vi "Supplementary Fig.15.vi"() -> ()   [LabVIEW 2018]
uses:
  <vilib>/Utility/miscctls.llb/LVBoundsTypeDef.ctl
  <vilib>/Analysis/baseanly.llb/Mean (DBL).vi
  <vilib>/Analysis/NI_AALBase.lvlib
panel:
  out "files":string[](array[string])=["3rd-no3_th0_20191112171700-ext.FIRE", "3rd-no3_th0_20191112171706-ext.FIRE", "3rd-no3_th0_20191112171712-ext.FIRE", "3rd-no3_th0_20191112171717-ext.FIRE", "3rd-no3_th0_20191112171723-ext.FIRE", "3rd-no3_th0_20191112171728-ext.FIRE", "3rd-no3_th0_20191112171733-ext.FIRE", "3rd-no3_th0_20191112171739-ext.FIRE", "3rd-no3_th0_20191112171744-ext.FIRE", "3rd-no3_th0_20191112171750-ext.FIRE", "3rd-no3_th0_20191112171756-ext.FIRE", "3rd-no3_th0_20191112171801-ext.FIRE", "3rd-no3_th0_20191112171807-ext.FIRE", "3rd-no3_th0_20191112171813-ext.FIRE", "3rd-no3_th0_20191112171819-ext.FIRE", "3rd-no3_th0_20191112171824-ext.FIRE", "3rd-no3_th0_20191112171829-ext.FIRE", "3rd-no3_th0_20191112171835-ext.FIRE", "3rd-no3_th0_20191112171840-ext.FIRE", "3rd-no3_th0_20191112171846-ext.FIRE", "3rd-no3_th0_20191112171851-ext.FIRE", "3rd-no3_th0_20191112171857-ext.FIRE"]
  in  "show imgs":bool=TRUE
  out "current frame":i32=701
  out "N of files":i32=22
  out "N of frames":i32=702
  out "current file index":i32=21
  in  "file type":string=".FIRE"
  in  "review all files":bool=TRUE
  in  "filepath":path
  out "appended path":path
  out "radius ch2y [pixels]":dbl=0.8053350059063624
  out "radius ch2x [pixels]":dbl=0.8398677103385433
  out "radius ch1y [pixels]":dbl=1.0235673529365912
  out "radius ch1x [pixels]":dbl=0.967080835109182
  out "ch1y":dbl[][](graph)=[[94.84941146149693, 94.84941146149693, 94.84941146149693, 94.84941146149693, 94.84941146149693, 94.84941146149693, 94.84941146149693, 94.84941146149693, 94.84941146149693, 94.84941146149693, 94.84941146149693, 94.84941146149693, 94.84941146149693, 94.84941146149693, 94.84941146149693, 94.84941146149693, 94.84941146149693, 94.84941146149693, 94.84941146149693, 94.84941146149693, 94.84941146149693, 94.84941146149693, 94.84941146149693, 94.84941146149693, 94.84941146149693, 94.84941146149693, 94.84941146149693, 94.84941146149693, 94.84941146149772, 94.84941146185378, 94.84941154507113, 94.84942162670632, 94.85005358097287, 94.87047691374316, 95.20831782861478, 98.02516630818968, 109.44320531116301, 129.67872185900958, 138.01890715732344, 122.63787314903747, 104.13923505734425, 96.46230558549654, 94.99484336321392, 94.85622180374438, 94.84957708944552, 94.84941355345867, 94.8494114752193, 94.84941146154368, 94.84941146149701, 94.84941146149693, 94.84941146149693, 94.84941146149693, 94.84941146149693, 94.84941146149693, 94.84941146149693, 94.84941146149693, 94.84941146149693, 94.84941146149693, 94.84941146149693, 94.84941146149693, 94.84941146149693, 94.84941146149693, 94.84941146149693, 94.84941146149693, 94.84941146149693, 94.84941146149693, 94.84941146149693, 94.84941146149693, 94.84941146149693, 94.84941146149693, 94.84941146149693, 94.84941146149693, 94.84941146149693, 94.84941146149693, 94.84941146149693, 94.84941146149693, 94.84941146149693, 94.84941146149693, 94.84941146149693, 94.84941146149693, 94.84941146149693, 94.84941146149693, 94.84941146149693, 94.84941146149693, 94.84941146149693, 94.84941146149693, 94.84941146149693, 94.84941146149693], [94.5, 101.0, 96.75, 88.5, 96.0, 90.0, 105.0, 87.0, 85.75, 86.5, 95.75, 98.75, 95.0, 98.0, 95.25, 89.75, 92.25, 93.5, 96.25, 101.75, 94.75, 93.75, 97.5, 96.75, 102.5, 93.5, 95.0, 94.25, 93.75, 91.5, 96.5, 96.75, 99.0, 93.75, 93.75, 100.5, 111.75, 125.25, 142.25, 120.25, 103.25, 99.5, 99.75, 96.75, 96.25, 96.5, 96.25, 95.5, 90.5, 94.5, 90.75, 93.75, 89.5, 92.5, 96.5, 96.5, 93.75, 99.25, 88.5, 93.75, 95.0, 93.5, 96.0, 97.0, 97.75, 96.25, 87.0, 93.25, 96.75, 95.25, 98.25, 95.25, 89.5, 96.75, 94.25, 101.5, 103.25, 98.25, 89.5, 90.75, 85.75, 100.5, 89.25, 94.5, 94.25, 94.25, 98.0, 96.5]]
  out "ch1x":dbl[][](graph)=[[95.60099317421837, 95.60099317421837, 95.60099317421837, 95.60099317421837, 95.60099317421837, 95.60099317421847, 95.60099317423827, 95.60099317665532, 95.60099336512587, 95.60100274141283, 95.60129988613946, 95.60728332652043, 95.6835163847676, 96.29358206377161, 99.31942115843458, 108.37207475424778, 123.6605258248726, 135.03924332581664, 131.06103889703965, 115.99701157117, 103.10573832119815, 97.36748223421115, 95.86698629539234, 95.62661524984625, 95.60257203072726, 95.60105541219495, 95.60099474368728, 95.60099319953666, 95.60099317447965, 95.6009931742201, 95.60099317421839, 95.60099317421837, 95.60099317421837, 95.60099317421837, 95.60099317421837, 95.60099317421837, 95.60099317421837, 95.60099317421837, 95.60099317421837, 95.60099317421837], [98.25, 92.75, 94.0, 97.0, 96.75, 95.25, 92.0, 94.0, 93.0, 95.25, 97.75, 95.25, 99.5, 96.0, 102.0, 111.0, 117.75, 138.75, 132.75, 110.25, 106.75, 101.5, 92.25, 98.5, 93.5, 93.75, 94.0, 96.25, 94.25, 95.75, 94.75, 97.75, 96.25, 95.0, 97.0, 95.5, 94.75, 94.0, 93.5, 100.0]]
  in  "parameter bounds":T1={"amp min"=0.0, "amp max"=70000.0, "center min"=5.0, "center max"=83.0, "deviation min"=0.0, "deviation max"=40.0, "offset min"=-100.0, "offset max"=1500.0}
  out "cy2x":dbl[][](graph)=[[94.12260003726622, 94.12260003726622, 94.12260003726622, 94.12260003726622, 94.12260003726622, 94.12260003726622, 94.12260003726622, 94.1226000372663, 94.12260003728049, 94.12260003914064, 94.12260019170165, 94.12260801439564, 94.12285836120417, 94.12784449955768, 94.18935069986297, 94.65523355745113, 96.78712447104466, 102.47919242915862, 110.55333652673302, 114.3762426102233, 109.77451759485643, 101.70576076839414, 96.42590408220602, 94.56120200791217, 94.17496106791177, 94.12651893647144, 94.12278391887723, 94.1226054464384, 94.12260013702281, 94.1226000384196, 94.12260003727458, 94.12260003726627, 94.12260003726622, 94.12260003726622, 94.12260003726622, 94.12260003726622, 94.12260003726622, 94.12260003726622, 94.12260003726622, 94.12260003726622], [90.75, 94.75, 94.5, 95.75, 96.5, 94.5, 95.25, 94.0, 92.75, 95.25, 95.5, 95.0, 92.75, 95.5, 98.0, 96.25, 94.25, 103.25, 110.75, 114.25, 109.75, 101.25, 97.25, 95.75, 94.25, 95.25, 96.0, 92.75, 93.0, 92.5, 93.0, 92.75, 95.0, 95.0, 92.5, 90.5, 92.25, 92.5, 93.0, 95.5]]
  out "ch2y":dbl[][](graph)=[[94.41876322918748, 94.41876322918748, 94.41876322918748, 94.41876322918748, 94.41876322918748, 94.41876322918748, 94.41876322918748, 94.41876322918748, 94.41876322918748, 94.41876322918748, 94.41876322918748, 94.41876322918748, 94.41876322918748, 94.41876322918748, 94.41876322918748, 94.41876322918748, 94.41876322918748, 94.41876322918748, 94.41876322918748, 94.41876322918748, 94.41876322918748, 94.41876322918748, 94.41876322918748, 94.41876322918748, 94.41876322918748, 94.41876322918748, 94.41876322918748, 94.41876322918748, 94.41876322918748, 94.41876322918748, 94.4187632292011, 94.41876326696479, 94.41879179174117, 94.42465132770943, 94.74971528540863, 99.49062116778822, 115.61120793579937, 118.56264068507656, 101.91848166532853, 95.05394040052857, 94.43343075240026, 94.41885557786252, 94.41876338771932, 94.41876322926167, 94.41876322918749, 94.41876322918748, 94.41876322918748, 94.41876322918748, 94.41876322918748, 94.41876322918748, 94.41876322918748, 94.41876322918748, 94.41876322918748, 94.41876322918748, 94.41876322918748, 94.41876322918748, 94.41876322918748, 94.41876322918748, 94.41876322918748, 94.41876322918748, 94.41876322918748, 94.41876322918748, 94.41876322918748, 94.41876322918748, 94.41876322918748, 94.41876322918748, 94.41876322918748, 94.41876322918748, 94.41876322918748, 94.41876322918748, 94.41876322918748, 94.41876322918748, 94.41876322918748, 94.41876322918748, 94.41876322918748, 94.41876322918748, 94.41876322918748, 94.41876322918748, 94.41876322918748, 94.41876322918748, 94.41876322918748, 94.41876322918748, 94.41876322918748, 94.41876322918748, 94.41876322918748, 94.41876322918748, 94.41876322918748, 94.41876322918748], [95.75, 98.5, 94.0, 93.25, 96.0, 94.5, 104.0, 87.75, 86.75, 88.0, 98.25, 100.75, 96.5, 91.25, 95.75, 90.25, 97.75, 94.0, 94.75, 101.0, 94.25, 88.25, 92.75, 88.25, 100.5, 94.5, 94.0, 97.0, 90.0, 90.5, 100.0, 92.0, 97.0, 97.0, 90.75, 97.25, 117.5, 117.0, 103.0, 98.75, 95.5, 100.0, 96.25, 95.75, 94.25, 93.25, 97.75, 91.5, 89.75, 94.0, 90.75, 94.0, 89.75, 93.75, 94.75, 95.5, 91.0, 95.5, 90.25, 95.25, 95.5, 90.75, 100.0, 94.5, 95.0, 96.5, 90.25, 91.0, 97.75, 97.5, 97.5, 95.0, 87.25, 98.25, 92.25, 95.25, 102.5, 93.25, 91.25, 92.5, 91.25, 102.5, 88.5, 95.75, 91.25, 94.75, 97.25, 95.25]]
  in  "Threshold Limits 2":cluster{"Lower value":sgl, "Upper value":sgl}={"Lower value"=20.0, "Upper value"=60005.0} {"Upper value" format="%.2f"; "Lower value" format="%.2f"}
  in  "Threshold Limits":cluster{"Lower value":sgl, "Upper value":sgl}={"Lower value"=50.0, "Upper value"=60000.0} {"Upper value" format="%.2f"; "Lower value" format="%.2f"}
  in  "input 2":T2={"Niblack Dev Fac"=0.6000000000000001, "Window"={"Width"=50, "Height"=50}, "Sauvola Dev Rng"=2.0, "adaptive"=FALSE, "Method (Niblack)"=1} {"Method (Niblack)" items=["Niblack", "Background Correction", "Sauvola"]}
  in  "in1":T2={"Niblack Dev Fac"=0.5, "Window"={"Width"=20, "Height"=20}, "Sauvola Dev Rng"=6000.0, "adaptive"=FALSE, "Method (Niblack)"=0} {"Method (Niblack)" items=["Niblack", "Background Correction", "Sauvola"]}
  in  "post proc 2":T3={"trunc for ch2 masking"=[2, 2, 5, 2], "Erosion(pre)"=2, "Op"=enum."PClose", "post proc"=TRUE, "move x/y"=[0, 0], "conv"=FALSE, "Conn"=TRUE, "iterations"=5, "Erosion(post)"=2}
  in  "post proc1":T4={"trunc for ch2 masking"=[0, 0, 0, 0], "Erosion(pre)"=2, "Op"=enum."PClose", "post proc"=FALSE, "move x/y"=[0, 0], "conv"=TRUE, "Conn"=TRUE, "iteration"=5, "Erosion(post)"=2}
  in  "seg meth 2":T5={"norm for thresh"=TRUE, "use thresh formula"=FALSE, "thresh"=0.27000000000000013, "man thresh"=FALSE, "Meth"=0, "upper lim"=65000} {"Meth" items=["clustering", "entropy", "metric", "moments", "inter-class variance"]; "thresh" format="%_3g"}
  in  "seg meth":T5={"norm for thresh"=TRUE, "use thresh formula"=FALSE, "thresh"=0.2999999999995926, "man thresh"=TRUE, "Meth"=0, "upper lim"=64100} {"Meth" items=["clustering", "entropy", "metric", "moments", "inter-class variance"]; "thresh" format="%_3g"}
  in  "lpf 2":cluster{"cut":dbl, "lpf":bool, "odr":i32}={"cut"=0.2900001, "lpf"=FALSE, "odr"=2} {"cut" min=1e-07 max=0.4999 step=0.01 format="%_2g"}
  in  "lpf 1":cluster{"cut":dbl, "lpf":bool, "odr":i32}={"cut"=0.15000010000000014, "lpf"=FALSE, "odr"=2} {"cut" min=1e-07 max=0.4999 step=0.01 format="%_2g"}
  in  "save data":bool=TRUE
  in  "scale fac1":dbl=1.0000000000000009 min=0.01 max=10.0 step=0.01 format="%_3g"
  in  "scale fac2":dbl=0.9999999999999983 min=0.01 max=10.0 step=0.01 format="%_3g"
  in  "autoscale":bool=TRUE
  out "ch1":picture
  out "ch2":picture
  in  "color":T6(array[cluster])=[{"color array"=[0, 16711680, 16776960, 16448250, 65280, 16776960, 16711680, 16448250, 16448250], "num of colors"=2, "max"=180.0, "min"=100.0}, {"color array"=[0, 65280, 16776960, 16448250, 65280, 16776960, 16711680, 16448250, 16448250], "num of colors"=2, "max"=9000.0, "min"=100.0}, {"color array"=[0, 255, 16448250, 16448250, 16776960, 16711680, 16448250, 16448250], "num of colors"=2, "max"=1.0, "min"=0.0}] {"min" step=0.01 format="%_2f"; "max" step=0.1 format="%_3f"}
  out "max2":dbl=185.0
  out "max1":dbl=216.0
  in  "Draw Area Size":T7
  in  "zoom":dbl=1.9999999999999973 format="%_2g"
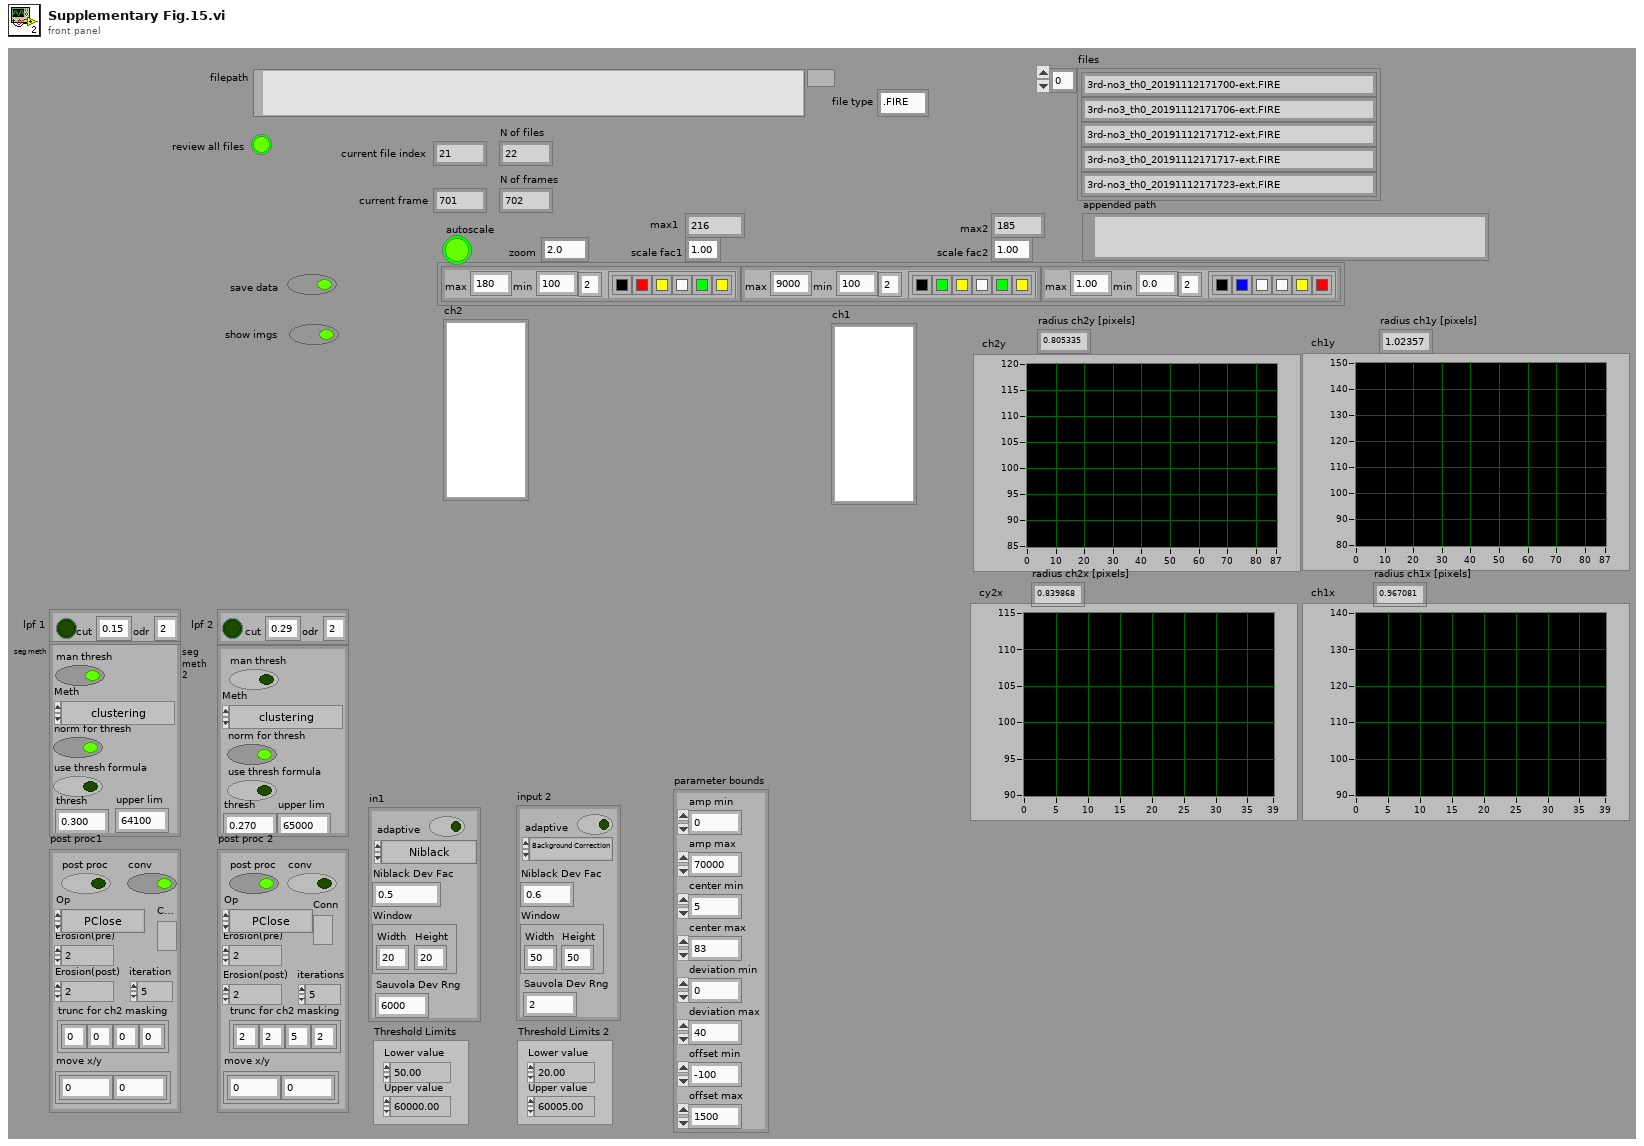
[diagram p1: front panel]
types:
  T1 = cluster{"amp min":dbl, "amp max":dbl, "center min":dbl, "center max":dbl, "deviation min":dbl, "deviation max":dbl, "offset min":dbl, "offset max":dbl}
  T2 = cluster{"Niblack Dev Fac":dbl, "Window":cluster{"Width":i32, "Height":i32}, "Sauvola Dev Rng":dbl, "adaptive":bool, "Method (Niblack)":u32}
  T3 = cluster{"trunc for ch2 masking":i32[], "Erosion(pre)":i32, "Op":enum32{"AutoM", "Close", "Dilate", "Erode", "Gradient", "Gradient out", "Gradient in", "Hit miss", "Open", "PClose", "POpen", "Thick", "Thin"}, "post proc":bool, "move x/y":i32[], "conv":bool, "Conn":bool, "iterations":i32, "Erosion(post)":i32}
  T4 = cluster{"trunc for ch2 masking":i32[], "Erosion(pre)":i32, "Op":enum32{"AutoM", "Close", "Dilate", "Erode", "Gradient", "Gradient out", "Gradient in", "Hit miss", "Open", "PClose", "POpen", "Thick", "Thin"}, "post proc":bool, "move x/y":i32[], "conv":bool, "Conn":bool, "iteration":i32, "Erosion(post)":i32}
  T5 = cluster{"norm for thresh":bool, "use thresh formula":bool, "thresh":dbl, "man thresh":bool, "Meth":i32, "upper lim":i32}
  T6 = cluster{"color array":u32[], "num of colors":i32, "max":dbl, "min":dbl}[]
  T7 = typedef "LVBoundsTypeDef.ctl" = cluster{"Width":u32, "Height":u32}
  T8 = enum16{"open", "replace", "create", "open or create", "replace or create", "replace or create with confirmation"}
  T9 = cluster{"color array":u32[], "num of colors":i32, "max":dbl, "min":dbl}
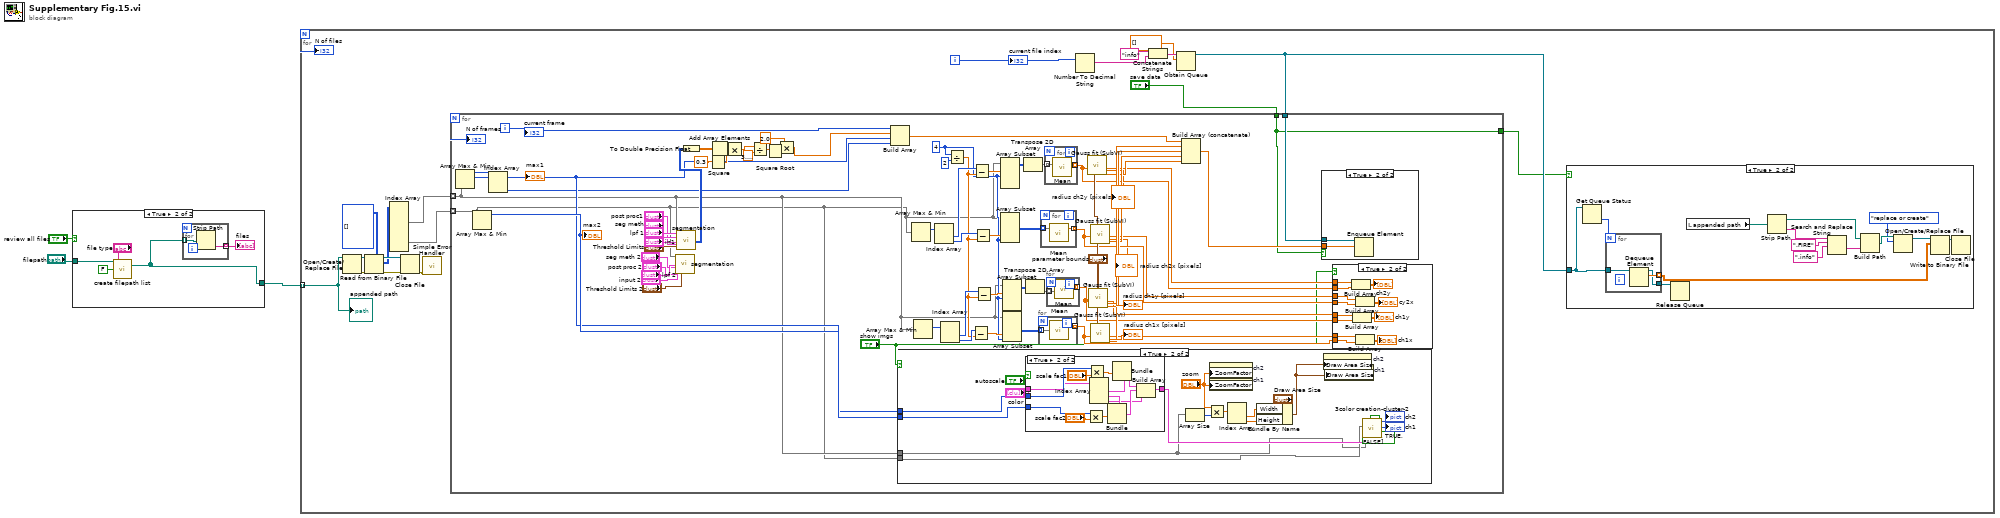
[diagram p0: block diagram]
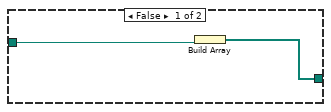
[diagram p2: hidden frame]
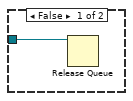
[diagram p7: hidden frame]
diagram:
  n1 = case shown="True" "review all files" {
    tunnel: "filepath" -> [w5 w8]
    tunnel: [w4 w7] -> w1
    frame False {
      n2 = Build Array(w5) -> (w4:path[])
    }
    frame True {
      n3 = call "create filepath list.vi"("regular expression"="file type", "search subholder"=FALSE, "path"=w8) -> ("Array"=w7:path[])  [unwired: 1 out]
      n4 = for {
        tunnel: w7 -> [w12] mode=indexing
        tunnel: [w11] -> w6 mode=indexing
        n5 = Strip Path(path=w12) -> (name=w11:string)  [unwired: 1 out]
      }
      "files" <- w6
    }
  }
  n6 = for {
    N -> [w13]
    tunnel: w1 -> [w19] mode=indexing
    i -> [w16]
    n7 = Open/Create/Replace File(file path (use dialog)=w19) -> (refnum out=w22:refnum<file>, error out=w23:errorcluster)  [unwired: 5 in, 1 out]
    n8 = Read from Binary File(5:i32[][][][] [], 8:w23, 11:w22) -> (0:w25:errorcluster, 2:w21:i32[][][][], 3:w26:refnum<file>)  [unwired: 3 in, 1 out]
    n9 = Index Array(array=w21) -> (element #1=w18:i32[][][], element #2=w17:i32[][][])  [unwired: 8 in]
    n10 = Close File(refnum=w26, error in=w25) -> (error out=w24:errorcluster)  [unwired: 1 out]
    n11 = call <vilib>:"Simple Error Handler.vi"("error in (no error)"=w24) -> ()  [unwired: 4 in, 5 out]
    n12 = Number To Decimal String(number=w16) -> (decimal integer string=w28:string)  [unwired: 1 in]
    n13 = Concatenate Strings("info" ("name (unnamed)"), w28) -> (w29:string)
    n14 = Obtain Queue(name (unnamed)=w29, element data type=dbl[] [] ("Array")) -> (queue out=w30:refnum<queue>)  [unwired: 3 in, 2 out]
    n15 = for {
      N -> [w34]
      tunnel: w30 -> [w90]
      tunnel: "save data" -> [w33]
      tunnel: w18 -> [w37] mode=indexing
      tunnel: w17 -> [w36] mode=indexing
      tunnel: [w33] -> w14
      i -> [w35]
      w57 = 4 ("y")
      n16 = Array Max & Min(array=w37) -> (max value=w78:i32, max index (indices)=w77:i32[])  [unwired: 2 out]
      "max1" <- w78
      n17 = Array Max & Min(array=w36) -> (max value=w93:i32)  [unwired: 3 out]
      "max2" <- w93
      n18 = Index Array(array=w77) -> (element #2=w76:i32)  [unwired: 2 in, 1 out]
      n19 = call "segmentation.vi"("unmixed ch2"=w36, "segmentation method"="seg meth 2", "image lpf"="lpf 2", "post processing"="post proc 2", "input cluster"="input 2", "Threshold Limits"="Threshold Limits 2") -> ()  [unwired: 7 in, 3 out]
      n20 = call "segmentation.vi"("unmixed ch2"=w37, "segmentation method"="seg meth", "image lpf"="lpf 1", "post processing"="post proc1", "input cluster"="in1", "Threshold Limits"="Threshold Limits") -> ("Array"=w89:u8[][])  [unwired: 7 in, 2 out]
      n21 = To Double Precision Float(number=w89) -> (double precision float=w80:dbl[][])
      n22 = Square(x=0.3) -> (x^2=w86:dbl)
      n23 = Add Array Elements(numeric array=w80) -> (sum=w88:dbl)
      n24 = Multiply(x=w88, y=w86) -> (x*y=w85:dbl)
      n25 = Divide(x=w85, y=3.141592653589793) -> (x/y=w83:dbl)
      n26 = Square Root(x=w83) -> (sqrt(x)=w82:dbl)
      n27 = Multiply(x=2.0, y=w82) -> (x*y=w79:dbl)
      n28 = Build Array(w35, w79, w78, w76) -> (w53:dbl[])
      n29 = case shown="True" "show imgs" {
        tunnel: w37 -> [_ w124]
        tunnel: w36 -> [_ w125]
        tunnel: w93 -> [_ w132]
        tunnel: w78 -> [_ w131]
        frame False {
        }
        frame True {
          n30 = case shown="True" "autoscale" {
            tunnel: w131 -> [_ w152]
            tunnel: w132 -> [_ w151]
            tunnel: "color" -> [w141 w148]
            tunnel: [w141 w147] -> w130
            frame False {
            }
            frame True {
              n31 = Multiply(x=w151, y="scale fac2") -> (x*y=w145:dbl)
              n32 = Multiply(x=w152, y="scale fac1") -> (x*y=w146:dbl)
              n33 = Index Array(array=w148) -> (element #1=w154:T9, element #2=w153:T9, element #3=w142:T9)  [unwired: 3 in]
              n34 = Bundle(cluster=w153, "max"=w145) -> (w149:T9)  [unwired: 3 in]
              n35 = Bundle(cluster=w154, "max"=w146) -> (w150:T9)  [unwired: 3 in]
              n36 = Build Array(w150, w149, w142) -> (w147:T6)
            }
          }
          n37 = Array Size(array=w124) -> (size(s)=w133:i32[])
          n38 = Multiply(x="zoom", y=w133) -> (x*y=w134:dbl[])
          n39 = property on="ch2" class="Pict"("ZoomFactor"="zoom") -> ()  [unwired: 2 in, 2 out]
          n40 = property on="ch1" class="Pict"("ZoomFactor"="zoom") -> ()  [unwired: 2 in, 2 out]
          n41 = Index Array(array=w134) -> (element #1=w126:dbl, element #2=w127:dbl)  [unwired: 2 in]
          n42 = Bundle By Name(cluster="Draw Area Size", "Width"=w126, "Height"=w127) -> (w137:T7)
          n43 = property on="ch2" class="Pict"("Draw Area Size"=w137) -> ()  [unwired: 2 in, 2 out]
          n44 = property on="ch1" class="Pict"("Draw Area Size"=w137) -> ()  [unwired: 2 in, 2 out]
          n45 = call "3color creation-cluster-2.vi"("color"=w130, "Array 4"=bool[] [TRUE, TRUE, FALSE], "Array 2"=w125, "Array"=w124) -> ("ch2"=→"ch1":picture, "ch1"=→"ch2":picture)  [unwired: 2 in, 2 out]
        }
      }
      n46 = Array Max & Min(array=w36) -> (max index (indices)=w75:i32[])  [unwired: 3 out]
      n47 = Array Max & Min(array=w37) -> (max index (indices)=w61:i32[])  [unwired: 3 out]
      n48 = Index Array(array=w75) -> (element #1=w67:i32, element #2=w70:i32)  [unwired: 2 in]
      n49 = Index Array(array=w61) -> (element #1=w60:i32, element #2=w59:i32)  [unwired: 2 in]
      n50 = Divide(x=w57, y=2) -> (x/y=w58:dbl)
      n51 = Subtract(x=w59, y=w58) -> (x-y=w64:dbl)
      n52 = Subtract(x=w67, y=w58) -> (x-y=w73:dbl)
      n53 = Subtract(x=w70, y=w58) -> (x-y=w71:dbl)
      n54 = Subtract(x=w60, y=w58) -> (x-y=w62:dbl)
      n55 = Array Subset(array=w36, index (row)=w73, length (row)=w57) -> (w69:i32[][])  [unwired: 2 in]
      n56 = Array Subset(array=w36, index (col)=w71, length (col)=w57) -> (w68:i32[][])  [unwired: 2 in]
      n57 = Array Subset(array=w37, index (row)=w62, length (row)=w57) -> (w65:i32[][])  [unwired: 2 in]
      n58 = Array Subset(array=w37, index (col)=w64, length (col)=w57) -> (w66:i32[][])  [unwired: 2 in]
      n59 = Transpose 2D Array(2D array=w69) -> (transposed array=w72:i32[][])
      n60 = Transpose 2D Array(2D array=w65) -> (transposed array=w63:i32[][])
      n61 = for {
        tunnel: w66 -> [w115] mode=indexing
        tunnel: [w114] -> w40 mode=indexing
        n62 = call-poly <vilib>:"Mean.vi"("X"=w115) -> ("mean"=w114:dbl)  [unwired: 1 out]
      }
      n63 = for {
        tunnel: w68 -> [w119] mode=indexing
        tunnel: [w118] -> w44 mode=indexing
        n64 = call-poly <vilib>:"Mean.vi"("X"=w119) -> ("mean"=w118:dbl)  [unwired: 1 out]
      }
      n65 = for {
        tunnel: w72 -> [w121] mode=indexing
        tunnel: [w120] -> w46 mode=indexing
        n66 = call-poly <vilib>:"Mean.vi"("X"=w121) -> ("mean"=w120:dbl)  [unwired: 1 out]
      }
      n67 = for {
        tunnel: w63 -> [w117] mode=indexing
        tunnel: [w116] -> w42 mode=indexing
        n68 = call-poly <vilib>:"Mean.vi"("X"=w117) -> ("mean"=w116:dbl)  [unwired: 1 out]
      }
      n69 = call "Gauss fit (SubVI).vi"("parameter bounds"="parameter bounds", "Array"=w46) -> ("results (a,c,s,r)"=w49:dbl[], "Best Gaussian Fit"=w47:dbl[], "standard deviation"=→"radius ch2y [pixels]":dbl)  [unwired: 4 in, 3 out]
      n70 = call "Gauss fit (SubVI).vi"("parameter bounds"="parameter bounds", "Array"=w42) -> ("results (a,c,s,r)"=w51:dbl[], "Best Gaussian Fit"=w43:dbl[], "standard deviation"=→"radius ch1y [pixels]":dbl)  [unwired: 4 in, 3 out]
      n71 = call "Gauss fit (SubVI).vi"("parameter bounds"="parameter bounds", "Array"=w40) -> ("results (a,c,s,r)"=w52:dbl[], "Best Gaussian Fit"=w41:dbl[], "standard deviation"=→"radius ch1x [pixels]":dbl)  [unwired: 4 in, 3 out]
      n72 = call "Gauss fit (SubVI).vi"("parameter bounds"="parameter bounds", "Array"=w44) -> ("results (a,c,s,r)"=w50:dbl[], "Best Gaussian Fit"=w45:dbl[], "standard deviation"=→"radius ch2x [pixels]":dbl)  [unwired: 4 in, 3 out]
      n73 = Build Array (concatenate)(w53, w52, w51, w50, w49) -> (w48:dbl[])
      n74 = case shown="True" w33 {
        tunnel: w90 -> [_ w123]
        tunnel: w48 -> [_ w122]
        frame False {
        }
        frame True {
          n75 = Enqueue Element(queue=w123, element=w122) -> ()  [unwired: 2 in, 3 out]
        }
      }
      n76 = case shown="True" "show imgs" {
        tunnel: w47 -> [_ w109]
        tunnel: w46 -> [_ w108]
        tunnel: w45 -> [_ w107]
        tunnel: w44 -> [_ w106]
        tunnel: w43 -> [_ w105]
        tunnel: w42 -> [_ w104]
        tunnel: w41 -> [_ w103]
        tunnel: w40 -> [_ w102]
        frame False {
        }
        frame True {
          n77 = Build Array(w109, w108) -> (→"ch2y":dbl[][])
          n78 = Build Array(w105, w104) -> (→"ch1y":dbl[][])
          n79 = Build Array(w103, w102) -> (→"ch1x":dbl[][])
          n80 = Build Array(w107, w106) -> (→"cy2x":dbl[][])
        }
      }
      "N of frames" <- w34
      "current frame" <- w35
    }
    n81 = case shown="True" w14 {
      tunnel: w30 -> [w155 w162]
      frame False {
        n82 = Release Queue(queue=w155) -> ()  [unwired: 2 in, 3 out]
      }
      frame True {
        n83 = Get Queue Status(queue=w162) -> (# elements in queue=w166:i32)  [unwired: 2 in, 7 out]
        n84 = for {
          N: w166 -> [_]
          tunnel: w162 -> [w172]
          tunnel: [w171] -> w161 mode=indexing
          tunnel: [w170] -> w165
          n85 = Dequeue Element(queue=w172) -> (queue out=w170:refnum<queue>, element=w171:dbl[])  [unwired: 2 in, 2 out]
        }
        n86 = Release Queue(queue=w165) -> ()  [unwired: 2 in, 3 out]
        n87 = local read "appended path"() -> (w158:path)
        n88 = Strip Path(path=w158) -> (stripped path=w156:path, name=w159:string)
        n89 = Search and Replace String(input string=w159, search string=".FIRE" ("substring (\"\")"), replace string=".info" ("replace string (\"\")")) -> (result string=w157:string)  [unwired: 5 in, 3 out]
        n90 = Build Path(base path=w156, name or relative path=w157) -> (appended path=w167:path)
        n91 = Open/Create/Replace File(file path (use dialog)=w167, operation (0:open)=T8."replace or create") -> (refnum out=w168:refnum<file>)  [unwired: 4 in, 2 out]
        n92 = Write to Binary File(file (use dialog)=w168, data=w161) -> (refnum out=w169:refnum<file>)  [unwired: 4 in, 2 out]
        n93 = Close File(refnum=w169) -> ()  [unwired: 1 in, 2 out]
      }
    }
    "appended path" <- w19
    "N of files" <- w13
    "current file index" <- w16
  }
